vi "Template Test - 24V.vi"(0 "Limits File Path":path, 5 "Results File Path":path, 11 "error in":errorcluster) -> (15 "error out":errorcluster)   [LabVIEW 2024]
doc: "Template test"
uses:
  <vilib>/addons/_JKI Toolkits/State Machine/_JKI_lib_State_Machine.llb/Select State(s)_err__jki_lib_state_machine.vi
  <userlib>/_OpenG.lib/file/file.llb/openg_file.lvlib
  <vilib>/Utility/file.llb/Read Delimited Spreadsheet (string).vi
  <userlib>/_OpenG.lib/file/file.llb/Strip Path Extension - String__ogtk.vi
  <userlib>/_OpenG.lib/appcontrol/appcontrol.llb/openg_application_control.lvlib
  <userlib>/_OpenG.lib/time/time.llb/openg_time.lvlib
  <vilib>/DAQmx/read.llb/DAQmx Read (Digital 1D Bool 1Chan 1Samp).vi
  <vilib>/DAQmx/create/channels.llb/DAQmx Create Channel (DI-Digital Input).vi
  <vilib>/addons/_JKI Toolkits/State Machine/_JKI_lib_State_Machine.llb/Select State(s)_bool__jki_lib_state_machine.vi
  <vilib>/Utility/file.llb/Write Delimited Spreadsheet (string).vi
panel:
  out "Timer Results Data":string[](array[string])
  out "24V Results Data":string[](array[string])
  in  "Exit":bool
  # "LED Test VI"
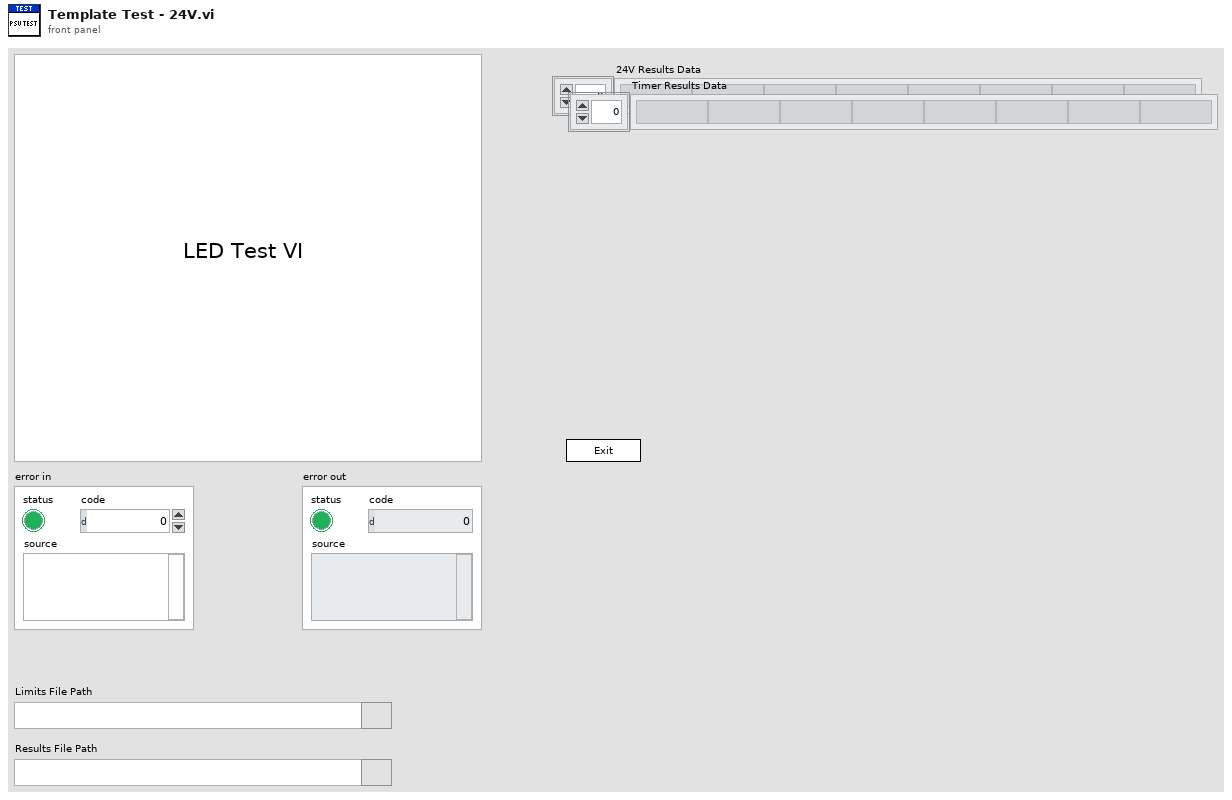
[diagram p1: front panel]
types:
  T1 = enum32{"Invalid", "Standard", "Closed", "Hidden", "Minimized", "Maximized"}
  T2 = enum32{"invalid app kind", "Development System", "Run Time System", "Student Edition", "Embedded LabVIEW", "Evaluation", "Custom"}
  T3 = enum16{"Start Timer", "Get Time", "Pause", "Unpause"}
  T4 = cluster{"Core":cluster{"Current VI Reference":refnum<vi>, "Close Panel on Exit?":bool}, "Limits File Path":path, "Test Limits":string[][], "Results Data Array":string[][], "Results File Path":path, "24V?":bool, "Time Elapsed?":bool, "task out":refnum<k21>}
  T5 = cluster{"Current VI Reference":refnum<vi>, "Close Panel on Exit?":bool}
  T6 = cluster{"[0]":bool, "[1]":bool, "[2]":bool, "[3]":bool, "[4]":bool, "[5]":bool, "[6]":bool, "[7]":bool, "[8]":bool}
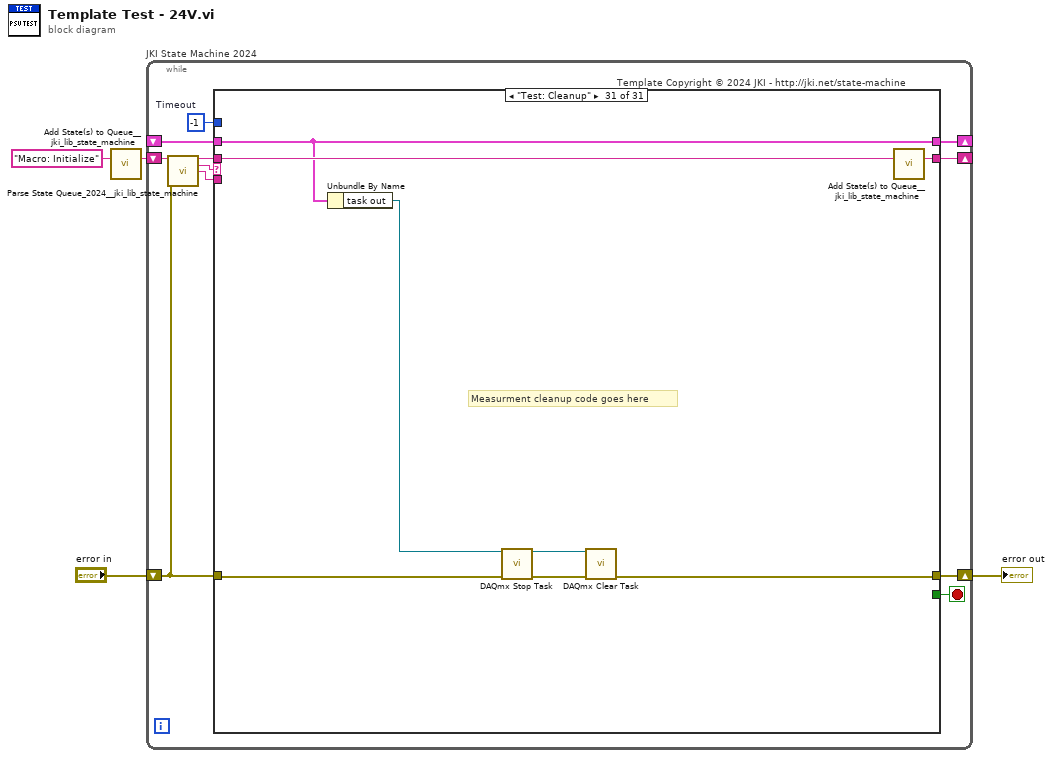
[diagram p0: block diagram]
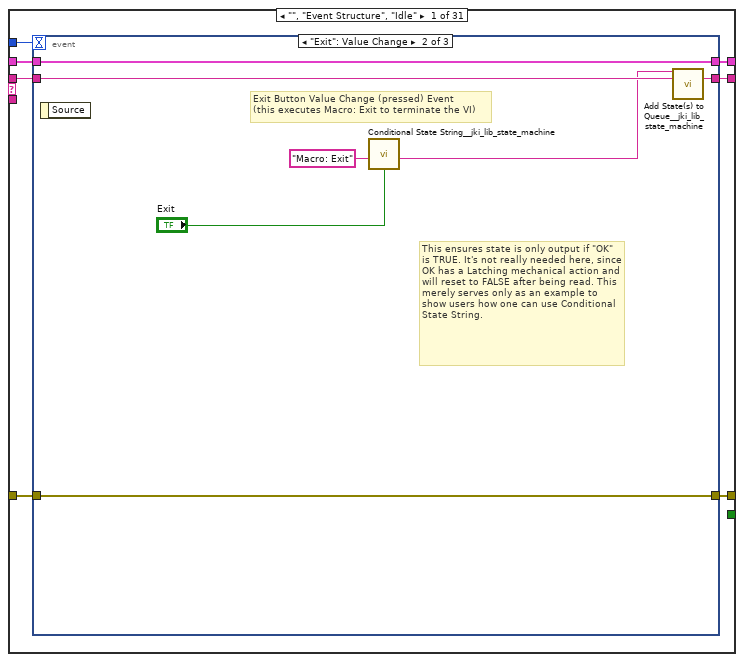
[diagram p2: hidden frame]
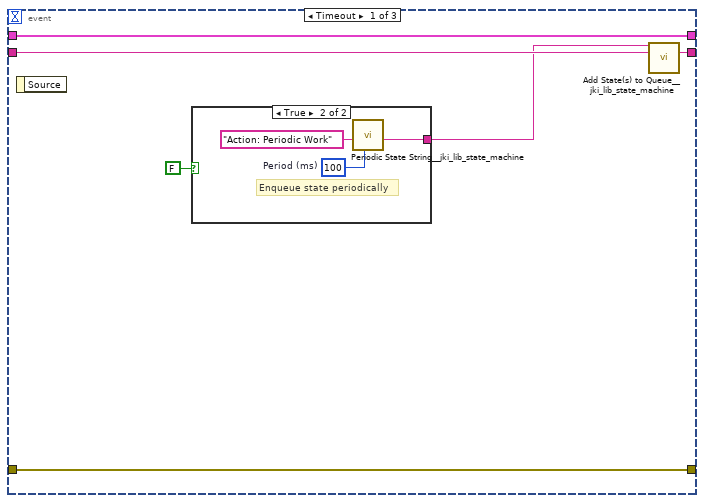
[diagram p3: hidden frame]
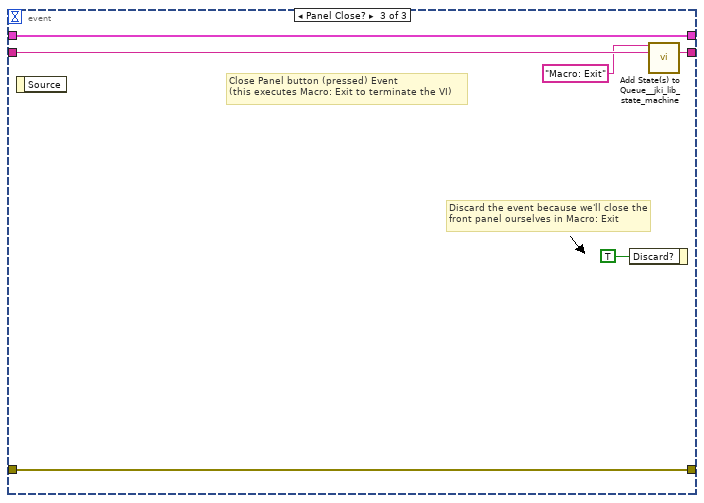
[diagram p5: hidden frame]
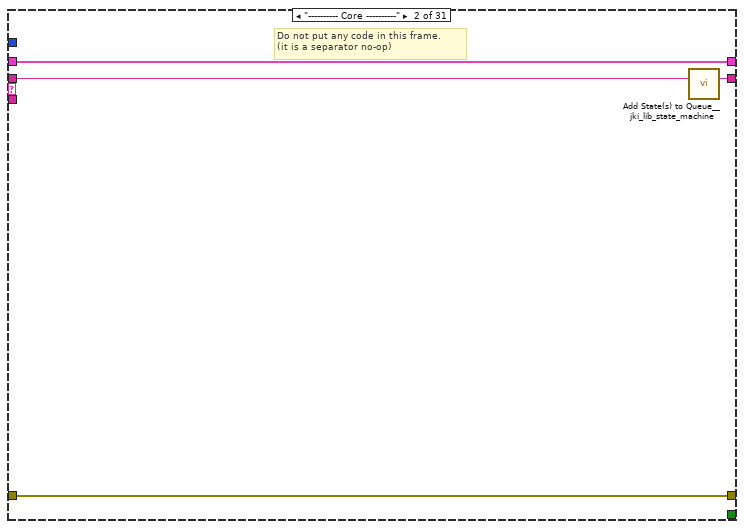
[diagram p6: hidden frame]
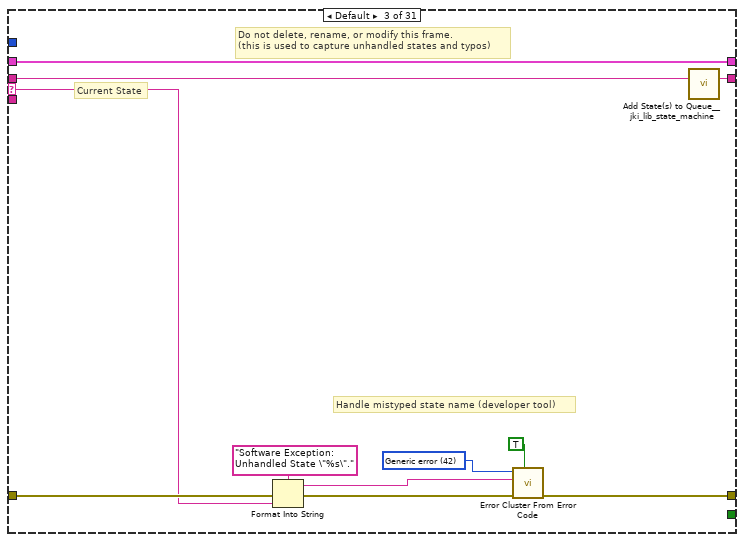
[diagram p7: hidden frame]
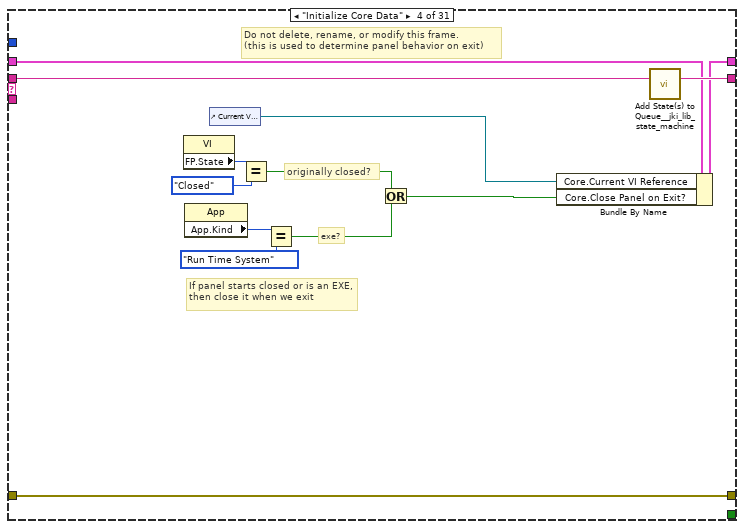
[diagram p8: hidden frame]
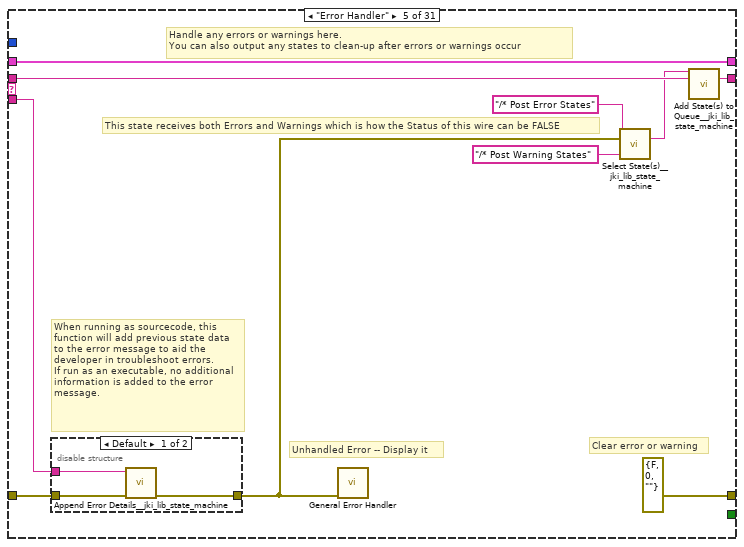
[diagram p9: hidden frame]
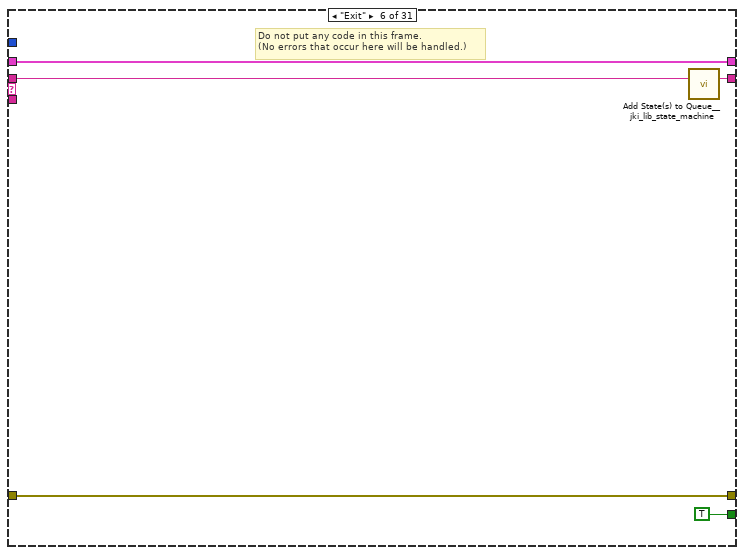
[diagram p11: hidden frame]
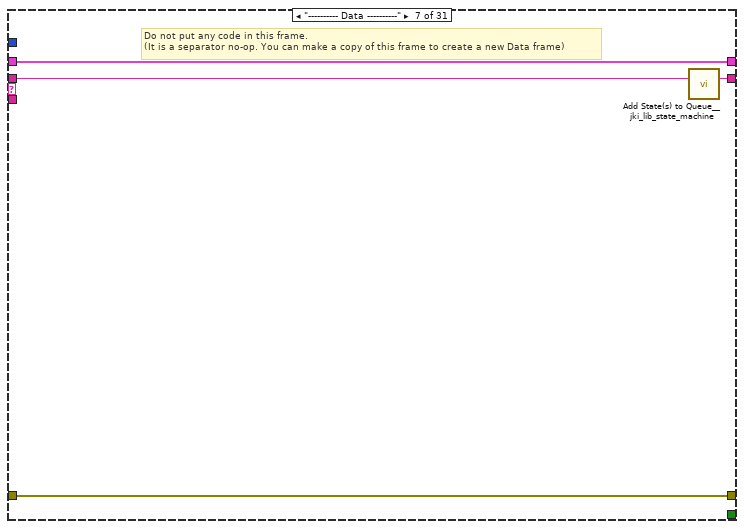
[diagram p12: hidden frame]
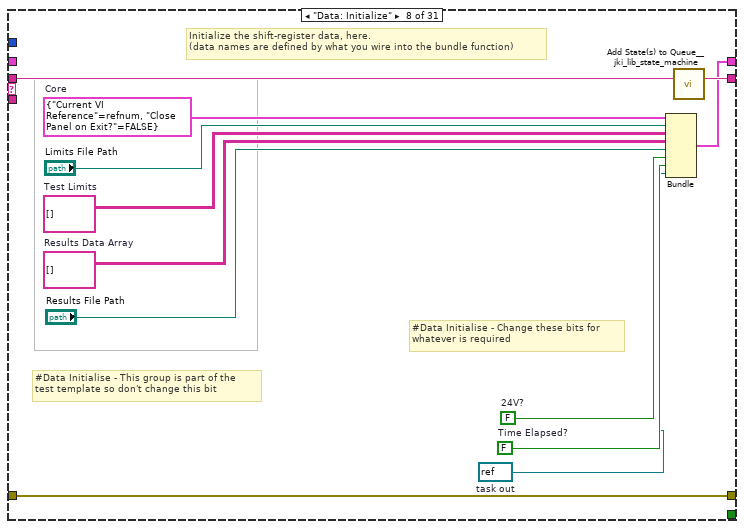
[diagram p13: hidden frame]
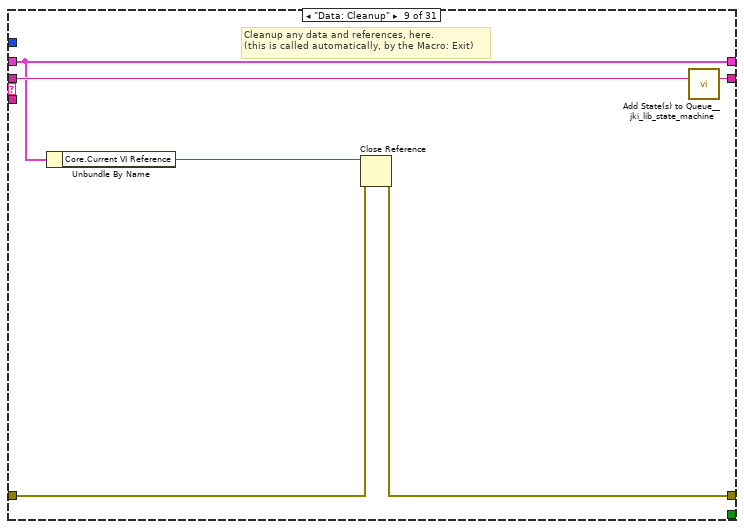
[diagram p14: hidden frame]
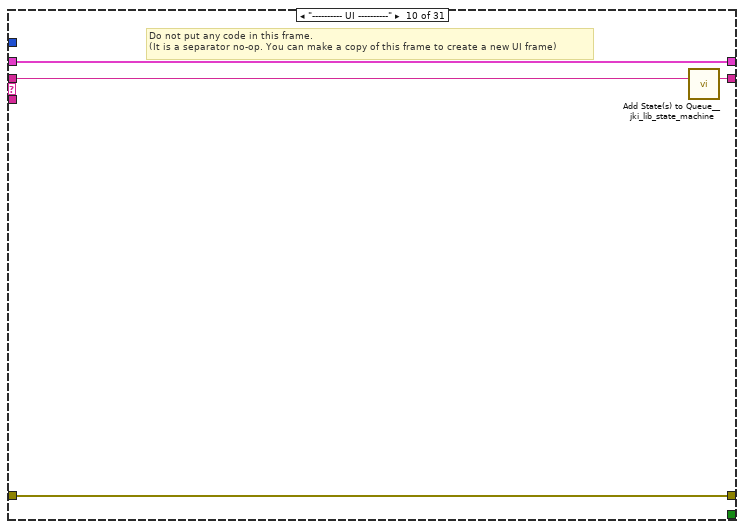
[diagram p15: hidden frame]
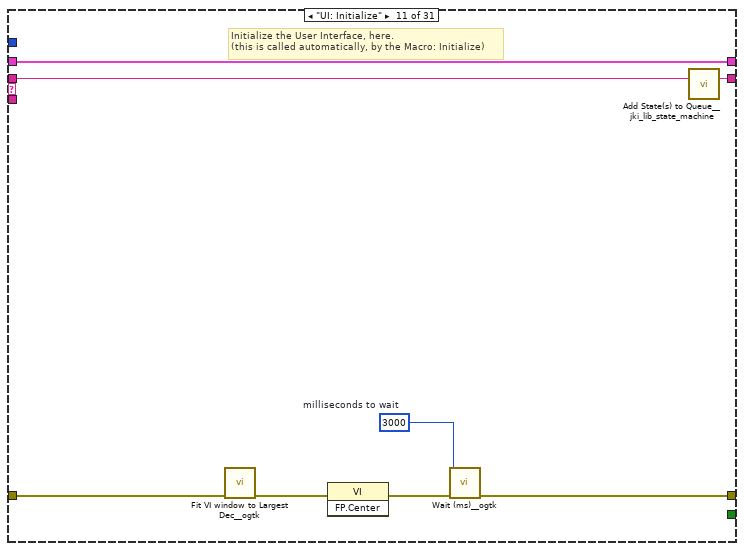
[diagram p16: hidden frame]
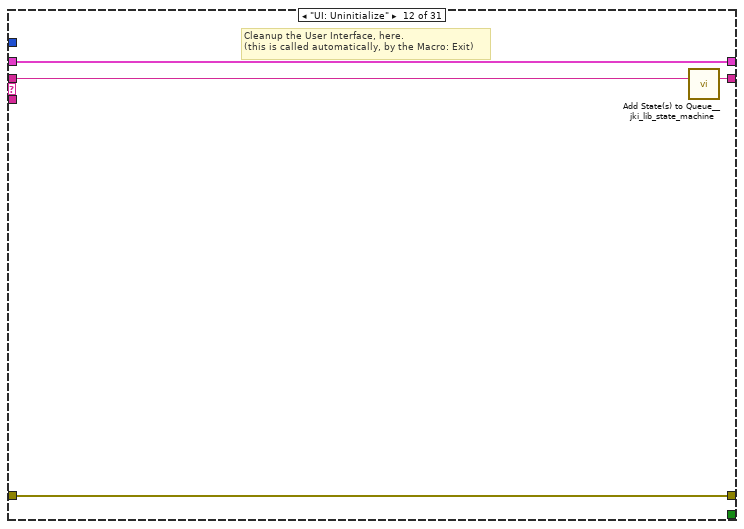
[diagram p17: hidden frame]
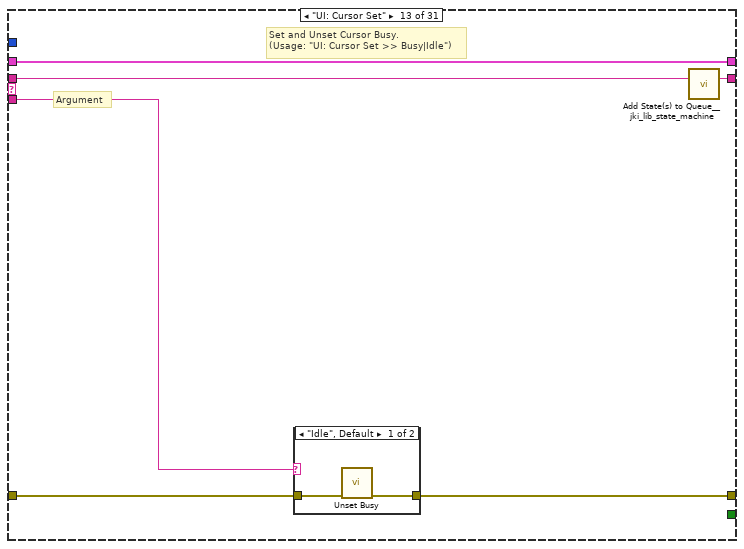
[diagram p18: hidden frame]
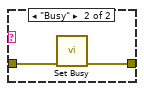
[diagram p19: hidden frame]
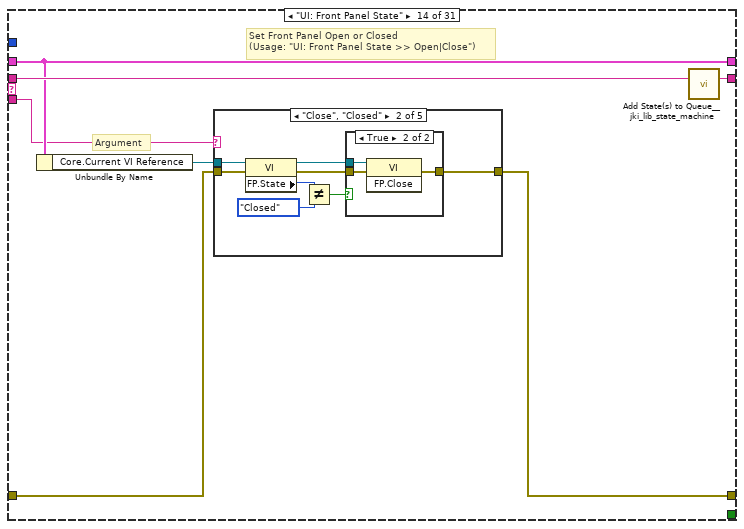
[diagram p20: hidden frame]
diagram:
  n1 = call <vilib>:"Add State(s) to Queue__jki_lib_state_machine.vi"("State(s) in (\"\")"="Macro: Initialize") -> ("States Out"=w4:string)  [unwired: 14 in]
  n2 = while "JKI State Machine 2024" {
    shift-right: [w8] -> _
    shift-left: _ -> [w7]
    shift-right: [w11] -> w1
    shift-left: "error in" -> [w5]
    shift-right: [w10] -> _
    shift-left: w4 -> [w12]
    stop <- w9 stop-if-true
    w6 = -1  # Timeout
    # "Template Copyright © 2024 JKI - http://jki.net/state-machine"
    n3 = call <vilib>:"Parse State Queue_2024__jki_lib_state_machine.vi"("State Queue"=w12, "Error In (no error)"=w5) -> ("Remaining States"=w14:string, "Current State"=w15:string, "Arguments"=w13:string)  [unwired: 11 in]
    n4 = case shown="\"Test: Cleanup\"" w15 {
      selector: w15 -> [_ _ w49 _ _ _ _ _ _ _ _ _ _ _ _ _ _ _ _ _ _ _ _ _ _ _ _ _ _ _ _]
      tunnel: w14 -> [w22 w48 w53 w72 w82 w91 w95 w107 w113 w117 w125 w129 w135 w146 w215 w220 w225 w230 w239 w243 w256 w273 w286 w290 w299 w303 w313 w319 w337 w349 w357]
      tunnel: w13 -> [_ _ _ _ w77 _ _ _ _ _ _ _ w130 w140 _ _ _ _ _ _ _ _ _ _ _ _ _ _ _ _ _]
      tunnel: w7 -> [w20 w45 w51 w65 w79 w89 w92 _ w108 w114 w123 w127 w133 w142 w212 w217 w222 w227 w237 w240 w246 w265 w278 w287 w295 w300 w306 w317 w321 w340 w351]
      tunnel: [w19 w46 w55 w69 errorcluster {"status"=FALSE, "code"=0, "source"=""} ("error out") w88 w93 w104 w109 w115 w121 w126 w131 w143 w213 w218 w223 w228 w234 w241 w252 w270 w283 w288 w297 w301 w307 w314 w326 w345 w353] -> w11
      tunnel: w5 -> [w16 w46 w54 w69 w78 w88 w93 w104 w110 w115 w122 w126 w132 w144 w213 w218 w223 w228 w234 w241 w251 w269 w282 w288 w296 w301 w308 w315 w329 w344 w352]
      tunnel: [w21 w47 w52 w71 w81 w90 w94 w106 w112 w116 w124 w128 w134 w145 w214 w219 w224 w229 w238 w242 w255 w272 w285 w289 w298 w302 w312 w318 w336 w348 w356] -> w10
      tunnel: [_ _ _ _ _ TRUE _ _ _ _ _ _ _ _ _ _ _ _ _ _ _ _ _ _ _ _ _ _ _ _ _] -> w9
      tunnel: [w18 w45 w51 w70 w79 w89 w92 w105 w108 w114 w123 w127 w133 w142 w212 w217 w222 w227 w237 w240 w245 w264 w277 w287 w295 w300 w305 w317 w335 w339 w351] -> w8
      tunnel: w6 -> [w17 _ _ _ _ _ _ _ _ _ _ _ _ _ _ _ _ _ _ _ _ _ _ _ _ _ _ _ _ _ _]
      frame "", "Event Structure", "Idle" {
        n5 = event shown="[1] \"Exit\": Value Change" {
          selector: _ -> [_ _ _]
          dyn-events: _ -> [_ _ _]
          timeout: w17 -> [_ _ _]
          tunnel: w22 -> [w28 w38 w44]
          tunnel: [w27 w37 w43] -> w21
          tunnel: w20 -> [w25 w35 w41]
          tunnel: [w26 w36 w42] -> w19
          tunnel: w16 -> [w26 w36 w42]
          tunnel: [w25 w35 w41] -> w18
          event Timeout {
            n6 = event-data() -> ()  [unwired: 1 in, 1 out]
            n7 = case shown="True" FALSE {
              tunnel: [_ w31] -> w24
              frame False {
              }
              frame True {
                w29 = u32 100  # Period (ms)
                # "Enqueue state periodically"
                n8 = call <vilib>:"Periodic State String__jki_lib_state_machine.vi"("Period (ms)"=w29, "State"="Action: Periodic Work") -> ("State Out"=w31:string)  [unwired: 9 in]
              }
            }
            n9 = call <vilib>:"Add State(s) to Queue__jki_lib_state_machine.vi"("State(s) in Front (\"\")"=w24, "State(s) in (\"\")"=w28) -> ("States Out"=w27:string)  [unwired: 13 in]
          }
          event "Exit": Value Change {
            # "This ensures state is only output if \"OK\" is TRUE. It's not really needed here, since OK has a Latching mechanical action and will reset to FALSE after being read. This merely serves only as an example to show users how one can use Conditional State String."
            # "Exit Button Value Change (pressed) Event\n(this executes Macro: Exit to terminate the VI)"
            n10 = event-data() -> ()  [unwired: 1 in, 1 out]
            n11 = call <vilib>:"Conditional State String__jki_lib_state_machine.vi"("Do State(s)?"="Exit", "State"="Macro: Exit") -> ("State Out"=w32:string)  [unwired: 7 in]
            n12 = call <vilib>:"Add State(s) to Queue__jki_lib_state_machine.vi"("State(s) in Front (\"\")"=w32, "State(s) in (\"\")"=w38) -> ("States Out"=w37:string)  [unwired: 13 in]
          }
          event Panel Close? {
            # "Discard the event because we'll close the front panel ourselves in Macro: Exit"
            # "Close Panel button (pressed) Event\n(this executes Macro: Exit to terminate the VI)"
            n13 = event-data() -> ()  [unwired: 1 in, 1 out]
            n14 = event-data("Discard?"=TRUE) -> ()  [unwired: 1 in, 1 out]
            n15 = call <vilib>:"Add State(s) to Queue__jki_lib_state_machine.vi"("State(s) in Front (\"\")"="Macro: Exit", "State(s) in (\"\")"=w44) -> ("States Out"=w43:string)  [unwired: 13 in]
          }
        }
      }
      frame "---------- Core ----------" {
        # "Do not put any code in this frame.\n(it is a separator no-op)"
        n16 = call <vilib>:"Add State(s) to Queue__jki_lib_state_machine.vi"("State(s) in (\"\")"=w48) -> ("States Out"=w47:string)  [unwired: 14 in]
      }
      frame Default {
        w58 = 42 items=["No error", "Argument error", "Memory is full", "Out of zone", "End of file", "File already open", "Generic file I/O error", "File not found", "File permission error", "Disk is full", "Duplicate path", "Too many files open", "System feature not enabled", "Resource file not found", "Cannot add resource", "Resource not found", "Image not found", "Image memory error", "Pen does not exist", "Config type invalid", "Config token not found", "Config parse error", "Config memory error", "Bad external code format", "Bad external code offset", "External code not present", "Null window", "Destroy window error", "Null menu", "Print aborted", "Bad print record", "Print driver error", "Windows error during printing", "Memory error during printing", "Print dialog error", "Generic print error", "Invalid device refnum", "Device not found", "Device parameter error", "Device unit error", "Cannot open device", "Device call aborted", "Generic error", "Cancelled by user", "Object ID too low", "Object ID too high", "Object not in heap", "Unknown heap", "Unknown object (invalid DefProc)", "Unknown object (DefProc not in table)", "Message out of range", "Invalid (null) method", "Unknown message", "Manager call not supported", "Bad address", "Network operation in progress", "Network operation timed out", "Connection is busy", "Network attribute not supported", "Network error", "Address in use", "System out of memory", "Connection aborted", "Connection refused", "Not connected", "Already connected", "Connection closed", "Initialization error (interapplication manager)", "Bad occurrence", "Wait on unbound occurrence handler", "Occurrence queue overflow", "Datalog type conflict", "Unused", "Unrecognized type (interapplication manager)", "Memory corrupt", "Failed to make temporary DLL", "Old CIN version", "Drag socket not found", "Failed to load drop-object", "Failed to register OLE object", "Failed to release OLE object", "Format specifier type mismatch", "Unknown format specifier", "Too few format specifiers", "Too many format specifiers", "Scan failed", "Newer CIN version", "Error converting to variant", "Runtime menu error", "Password tampered", "Variant attribute not found", "Incompatible variant data type", "Event data is not available", "Event Store is not present", "Occurrence is not found", "Event Queue is not created", "Event info is not available", "Refnum passed is NULL", "Error retrieving Class GUID", "Error retrieving CoClass GUID", "Error retrieving TypeLib GUID.", "Bad built application magic bytes.", "Specific driver is different from the specific driver associated with the Logical Name.", "There is no session opened to the class driver.", "Max Error", "MAX - Error with config objects", "MAX - Error loading configuration", "MAX - Group not supported"]
        # "Current State"
        # "Do not delete, rename, or modify this frame.\n(this is used to capture unhandled states and typos)"
        # "Handle mistyped state name (developer tool)"
        n17 = Format Into String(format string="Software Exception: Unhandled State \"%s\"." ("message"), error in=w54, w49) -> (resulting string=w57:string, error out=w56:errorcluster)  [unwired: 1 in]
        n18 = call <vilib>:"Error Cluster From Error Code.vi"("show call chain? (False)"=TRUE, "error in (no error)"=w56, "error message (\"\")"=w57, "error code (0)"=w58) -> ("error out"=w55:errorcluster)  [unwired: 5 in]
        n19 = call <vilib>:"Add State(s) to Queue__jki_lib_state_machine.vi"("State(s) in (\"\")"=w53) -> ("States Out"=w52:string)  [unwired: 14 in]
      }
      frame "Initialize Core Data" {
        # "Do not delete, rename, or modify this frame.\n(this is used to determine panel behavior on exit)"
        # "originally closed?"
        # "exe?"
        # "If panel starts closed or is an EXE, then close it when we exit"
        n20 = property class="VI"() -> ("FP.State"=w62:T1)  [unwired: 2 in, 2 out]
        n21 = property class="App"() -> ("App.Kind"=w68:T2)  [unwired: 2 in, 2 out]
        n22 = control-ref of="Current VI Reference"() -> (w63:refnum<vi>)
        n23 = Equal?(x=w62, y=T1."Closed" ("Front Panel Window:State")) -> (x = y?=w60:bool)
        n24 = Equal?(x=w68, y=T2."Run Time System" ("Application:Kind")) -> (x = y?=w66:bool)
        n25 = Or(x=w60, y=w66) -> (x .or. y?=w64:bool)
        n26 = Bundle By Name(cluster=w65, "Core.Current VI Reference"=w63, "Core.Close Panel on Exit?"=w64) -> (w70:T4)
        n27 = call <vilib>:"Add State(s) to Queue__jki_lib_state_machine.vi"("State(s) in (\"\")"=w72) -> ("States Out"=w71:string)  [unwired: 14 in]
      }
      frame "Error Handler" {
        # "When running as sourcecode, this function will add previous state data to the error message to aid the developer in troubleshoot errors.\nIf run as an executable, no additional information is added to the error message."
        # "This state receives both Errors and Warnings which is how the Status of this wire can be FALSE"
        # "Unhandled Error -- Display it"
        # "Handle any errors or warnings here.\nYou can also output any states to clean-up after errors or warnings occur"
        # "Clear error or warning"
        n28 = disable-structure shown="Default" {
          disable-tunnel: w78 -> [w85 w86]
          disable-tunnel: w77 -> [w84 _]
          disable-tunnel: [w83 w86] -> w76
          frame condition #0 (active) {
            n29 = call <vilib>:"Append Error Details__jki_lib_state_machine.vi"("error in (no error)"=w85, "Previous State and Argument(s)"=w84) -> ("error out"=w83:errorcluster)  [unwired: 9 in]
          }
          frame condition #1 {
          }
        }
        n30 = call <vilib>:"General Error Handler.vi"("error in (no error)"=w76) -> ()  [unwired: 10 in, 5 out]
        n31 = call-poly <vilib>:"Select State(s)__jki_lib_state_machine.vi"("State(s) if True (\"\")"="/* Post Error States", "Select"=w76, "State(s) if False (\"\")"="/* Post Warning States") -> ("States Out"=w74:string)  [unwired: 12 in]
        n32 = call <vilib>:"Add State(s) to Queue__jki_lib_state_machine.vi"("State(s) in Front (\"\")"=w74, "State(s) in (\"\")"=w82) -> ("States Out"=w81:string)  [unwired: 13 in]
      }
      frame "Exit" {
        # "Do not put any code in this frame.\n(No errors that occur here will be handled.)"
        n33 = call <vilib>:"Add State(s) to Queue__jki_lib_state_machine.vi"("State(s) in (\"\")"=w91) -> ("States Out"=w90:string)  [unwired: 14 in]
      }
      frame "---------- Data ----------" {
        # "Do not put any code in this frame.\n(It is a separator no-op. You can make a copy of this frame to create a new Data frame)"
        n34 = call <vilib>:"Add State(s) to Queue__jki_lib_state_machine.vi"("State(s) in (\"\")"=w95) -> ("States Out"=w94:string)  [unwired: 14 in]
      }
      frame "Data: Initialize" {
        w96 = refnum<k21> refnum  # task out
        w97 = FALSE  # Time Elapsed?
        w98 = FALSE  # 24V?
        w100 = string[][] []  # Results Data Array
        w101 = string[][] []  # Test Limits
        w103 = T5 {"Current VI Reference"=refnum, "Close Panel on Exit?"=FALSE}  # Core
        # "#Data Initialise - Change these bits for\nwhatever is required"
        # "#Data Initialise - This group is part of the\ntest template so don't change this bit"
        # "Initialize the shift-register data, here.\n(data names are defined by what you wire into the bundle function)"
        n35 = Bundle("Core"=w103, "Limits File Path"="Limits File Path", "Test Limits"=w101, "Results Data Array"=w100, "Results File Path"="Results File Path", "24V?"=w98, "Time Elapsed?"=w97, "task out"=w96) -> (w105:T4)  [unwired: 1 in]
        n36 = call <vilib>:"Add State(s) to Queue__jki_lib_state_machine.vi"("State(s) in (\"\")"=w107) -> ("States Out"=w106:string)  [unwired: 14 in]
      }
      frame "Data: Cleanup" {
        # "Cleanup any data and references, here.\n(this is called automatically, by the Macro: Exit)"
        n37 = Unbundle By Name(w108) -> ("Core.Current VI Reference"=w111:refnum<vi>)
        n38 = Close Reference(reference=w111, error in (no error)=w110) -> (error out=w109:errorcluster)
        n39 = call <vilib>:"Add State(s) to Queue__jki_lib_state_machine.vi"("State(s) in (\"\")"=w113) -> ("States Out"=w112:string)  [unwired: 14 in]
      }
      frame "---------- UI ----------" {
        # "Do not put any code in this frame.\n(It is a separator no-op. You can make a copy of this frame to create a new UI frame)"
        n40 = call <vilib>:"Add State(s) to Queue__jki_lib_state_machine.vi"("State(s) in (\"\")"=w117) -> ("States Out"=w116:string)  [unwired: 14 in]
      }
      frame "UI: Initialize" {
        w120 = u32 3000  # milliseconds to wait
        # "Initialize the User Interface, here.\n(this is called automatically, by the Macro: Initialize)"
        n41 = call <userlib>:"Fit VI window to Largest Dec__ogtk.vi"("error in (no error)"=w122) -> ("error out"=w118:errorcluster)  [unwired: 5 in, 1 out]
        n42 = invoke class="VI" method="FP.Center"(error in=w118) -> (error out=w119:errorcluster)  [unwired: 2 in, 2 out]
        n43 = call <userlib>:"Wait (ms)__ogtk.vi"("error in (no error)"=w119, "milliseconds to wait"=w120) -> ("error out"=w121:errorcluster)  [unwired: 8 in, 1 out]
        n44 = call <vilib>:"Add State(s) to Queue__jki_lib_state_machine.vi"("State(s) in (\"\")"=w125) -> ("States Out"=w124:string)  [unwired: 14 in]
      }
      frame "UI: Uninitialize" {
        # "Cleanup the User Interface, here.\n(this is called automatically, by the Macro: Exit)"
        n45 = call <vilib>:"Add State(s) to Queue__jki_lib_state_machine.vi"("State(s) in (\"\")"=w129) -> ("States Out"=w128:string)  [unwired: 14 in]
      }
      frame "UI: Cursor Set" {
        # "Argument"
        # "Set and Unset Cursor Busy.\n(Usage: \"UI: Cursor Set >> Busy|Idle\")"
        n46 = case shown="\"Idle\", Default" w130 {
          tunnel: w132 -> [w137 w139]
          tunnel: [w136 w138] -> w131
          frame "Idle", Default {
            n47 = call <vilib>:"Unset Busy.vi"("error in (no error)"=w137) -> ("error out"=w136:errorcluster)  [unwired: 10 in]
          }
          frame "Busy" {
            n48 = call <vilib>:"Set Busy.vi"("error in (no error)"=w139) -> ("error out"=w138:errorcluster)  [unwired: 9 in, 1 out]
          }
        }
        n49 = call <vilib>:"Add State(s) to Queue__jki_lib_state_machine.vi"("State(s) in (\"\")"=w135) -> ("States Out"=w134:string)  [unwired: 14 in]
      }
      frame "UI: Front Panel State" {
        # "Argument"
        # "Set Front Panel Open or Closed\n(Usage: \"UI: Front Panel State >> Open|Close\")"
        n50 = Unbundle By Name(w142) -> ("Core.Current VI Reference"=w141:refnum<vi>)
        n51 = case shown="\"Close\", \"Closed\"" w140 {
          tunnel: w144 -> [w152 w167 w178 w191 w204]
          tunnel: [w154 w168 w180 w193 w206] -> w143
          tunnel: w141 -> [w153 w165 w179 w192 w205]
          frame "Open", "Standard", Default {
            w147 = T1."Standard" ("State")
            n52 = property class="VI"(reference=w153, error in=w152) -> (reference out=w150:refnum<vi>, error out=w151:errorcluster, "FP.State"=w149:T1)
            n53 = Not Equal?(x=w149, y=w147) -> (x != y?=w148:bool)
            n54 = case shown="True" w148 {
              tunnel: [w158 w160] -> w154
              tunnel: w151 -> [w157 w160]
              tunnel: w150 -> [w156 _]
              tunnel: w147 -> [w155 _]
              frame True {
                n55 = invoke class="VI" method="FP.Open"(reference=w156, error in=w157, "Activate"=TRUE, "State"=w155) -> (error out=w158:errorcluster)  [unwired: 1 in, 4 out]
              }
              frame False {
              }
            }
          }
          frame "Close", "Closed" {
            n56 = property class="VI"(reference=w165, error in=w167) -> (reference out=w164:refnum<vi>, error out=w166:errorcluster, "FP.State"=w162:T1)
            n57 = Not Equal?(x=w162, y=T1."Closed" ("Front Panel Window:State")) -> (x != y?=w161:bool)
            n58 = case shown="True" w161 {
              tunnel: [w169 w172] -> w168
              tunnel: w166 -> [w169 w171]
              tunnel: w164 -> [_ w170]
              frame False {
              }
              frame True {
                n59 = invoke class="VI" method="FP.Close"(reference=w170, error in=w171) -> (error out=w172:errorcluster)  [unwired: 1 in, 2 out]
              }
            }
          }
          frame "Hidden", "Hide" {
            w173 = T1."Hidden" ("State")
            n60 = property class="VI"(reference=w179, error in=w178) -> (reference out=w176:refnum<vi>, error out=w177:errorcluster, "FP.State"=w175:T1)
            n61 = Not Equal?(x=w175, y=w173) -> (x != y?=w174:bool)
            n62 = case shown="True" w174 {
              tunnel: [w184 w185] -> w180
              tunnel: w177 -> [w183 w185]
              tunnel: w176 -> [w182 _]
              tunnel: w173 -> [w181 _]
              frame True {
                n63 = invoke class="VI" method="FP.Open"(reference=w182, error in=w183, "State"=w181) -> (error out=w184:errorcluster)  [unwired: 2 in, 4 out]
              }
              frame False {
              }
            }
          }
          frame "Minimize", "Minimized" {
            w186 = T1."Minimized" ("State")
            n64 = property class="VI"(reference=w192, error in=w191) -> (reference out=w189:refnum<vi>, error out=w190:errorcluster, "FP.State"=w188:T1)
            n65 = Not Equal?(x=w188, y=w186) -> (x != y?=w187:bool)
            n66 = case shown="True" w187 {
              tunnel: [w197 w198] -> w193
              tunnel: w190 -> [w196 w198]
              tunnel: w189 -> [w195 _]
              tunnel: w186 -> [w194 _]
              frame True {
                n67 = invoke class="VI" method="FP.Open"(reference=w195, error in=w196, "State"=w194) -> (error out=w197:errorcluster)  [unwired: 2 in, 4 out]
              }
              frame False {
              }
            }
          }
          frame "Maximize", "Maximized" {
            w199 = T1."Maximized" ("State")
            n68 = property class="VI"(reference=w205, error in=w204) -> (reference out=w202:refnum<vi>, error out=w203:errorcluster, "FP.State"=w201:T1)
            n69 = Not Equal?(x=w201, y=w199) -> (x != y?=w200:bool)
            n70 = case shown="True" w200 {
              tunnel: [w210 w211] -> w206
              tunnel: w203 -> [w209 w211]
              tunnel: w202 -> [w208 _]
              tunnel: w199 -> [w207 _]
              frame True {
                n71 = invoke class="VI" method="FP.Open"(reference=w208, error in=w209, "State"=w207) -> (error out=w210:errorcluster)  [unwired: 2 in, 4 out]
              }
              frame False {
              }
            }
          }
        }
        n72 = call <vilib>:"Add State(s) to Queue__jki_lib_state_machine.vi"("State(s) in (\"\")"=w146) -> ("States Out"=w145:string)  [unwired: 14 in]
      }
      frame "---------- Macro ----------" {
        # "Do not put any code in this frame.\n(It is a separator no-op. You can make a copy of this frame to create a new Macro frame)"
        n73 = call <vilib>:"Add State(s) to Queue__jki_lib_state_machine.vi"("State(s) in (\"\")"=w215) -> ("States Out"=w214:string)  [unwired: 14 in]
      }
      frame "Macro: Initialize" {
        # "Initialization Macro\n(This is called once, when the VI starts)"
        n74 = call <vilib>:"Add State(s) to Queue__jki_lib_state_machine.vi"("State(s) in Front (\"\")"="Data: Initialize\nInitialize Core Data\nUI: Initialize\nUI: Front Panel State >> Open\nMacro: Test", "State(s) in (\"\")"=w220) -> ("States Out"=w219:string)  [unwired: 13 in]
      }
      frame "Macro: Test" {
        # "#Test Macro - Add the sequence \nfor measurments and limits testing here"
        n75 = call <vilib>:"Add State(s) to Queue__jki_lib_state_machine.vi"("State(s) in Front (\"\")"="Test: Initialise\nTest: Start Timer\nTest: Measurment", "State(s) in (\"\")"=w225) -> ("States Out"=w224:string)  [unwired: 13 in]
      }
      frame "Macro: Limits" {
        # "#Test Macro - Add the sequence \nfor measurments and limits testing here"
        n76 = call <vilib>:"Add State(s) to Queue__jki_lib_state_machine.vi"("State(s) in Front (\"\")"="Limits Test: Read Limits File\nLimits Test: 24V Test\nLimits Test: Timer Elapsed\nMacro: Exit", "State(s) in (\"\")"=w230) -> ("States Out"=w229:string)  [unwired: 13 in]
      }
      frame "Macro: Exit" {
        # "Exit Macro\n(This is called once, when the VI exits)"
        n77 = Unbundle By Name(w237) -> ("Core.Close Panel on Exit?"=w232:bool)
        n78 = call <vilib>:"Conditional State String__jki_lib_state_machine.vi"("Do State(s)?"=w232, "State"="UI: Front Panel State >> Close") -> ("State Out"=w231:string)  [unwired: 7 in]
        n79 = call <vilib>:"Add State(s) to Queue__jki_lib_state_machine.vi"("State(s) in (\"\")"=w231, "State(s) at Back (\"\")"="Test: Cleanup\nUI: Uninitialize\nData: Cleanup\nExit") -> ("States Out"=w235:string)  [unwired: 13 in]
        n80 = call <vilib>:"Add State(s) to Queue__jki_lib_state_machine.vi"("State(s) in Front (\"\")"=w235, "State(s) in (\"\")"=w239) -> ("States Out"=w238:string)  [unwired: 13 in]
      }
      frame "---------- Limits Test ----------" {
        # "Template Separator\n(You can make a copy of, or modify, this frame)"
        n81 = call <vilib>:"Add State(s) to Queue__jki_lib_state_machine.vi"("State(s) in (\"\")"=w243) -> ("States Out"=w242:string)  [unwired: 14 in]
      }
      frame "Limits Test: Read Limits File" {
        w249 = ","  # delimiter (\t)
        n82 = Unbundle By Name(w246) -> ("Limits File Path"=w250:path)
        n83 = Current VI's Path "Test Case Path"() -> (path=w254:path)
        n84 = call-poly <vilib>:"Read Delimited Spreadsheet.vi"("file path (dialog if empty)"=w250, "error in (no error)"=w251, "delimiter (\\t)"=w249) -> ("all rows"=w247:string[][], "error out"=w252:errorcluster)  [unwired: 7 in, 4 out]
        n85 = Strip Path(path=w254) -> (name=w253:string)  [unwired: 1 out]
        n86 = call-poly <userlib>:"Strip Path Extension__ogtk.vi"("path"=w253) -> ("root"=w248:string)  [unwired: 1 out]
        n87 = for {
          tunnel: w248 -> [w260]
          tunnel: w247 -> [w258] mode=indexing
          tunnel: [w258] -> w244 mode=indexing if=w257
          n88 = Index Array(array=w258) -> (element=w259:string)  [unwired: 1 in]
          n89 = Equal?(x=w260, y=w259) -> (x = y?=w257:bool)
        }
        n90 = Bundle By Name(cluster=w246, "Test Limits"=w244) -> (w245:T4)
        n91 = call <vilib>:"Add State(s) to Queue__jki_lib_state_machine.vi"("State(s) in (\"\")"=w256) -> ("States Out"=w255:string)  [unwired: 14 in]
      }
      frame "Limits Test: 24V Test" {
        w266 = "24V Test"  # Sub Test Name
        # "#Limits Testing - Add the sub test name for\ntest included in limits file"
        n92 = Unbundle By Name(w265) -> ("Results Data Array"=w263:string[][])
        n93 = Unbundle By Name(w265) -> ("Test Limits"=w267:string[][], "24V?"=w271:bool)
        n94 = To Variant(anything=w271) -> (Variant=w268:variant)
        n95 = call "Process Results.vi"("error in (no error)"=w269, "Measurment"=w268, "Test Limits"=w267, "Sub Test Name"=w266) -> ("error out"=w270:errorcluster, "Results Data"=w262:string[])  [unwired: 6 in]
        "24V Results Data" <- w262
        n96 = Build Array (concatenate)(w263, w262) -> (w261:string[][])
        n97 = Bundle By Name(cluster=w265, "Results Data Array"=w261) -> (w264:T4)
        n98 = call <vilib>:"Add State(s) to Queue__jki_lib_state_machine.vi"("State(s) in (\"\")"=w273) -> ("States Out"=w272:string)  [unwired: 14 in]
      }
      frame "Limits Test: Timer Elapsed" {
        w279 = "TimerTest"  # Sub Test Name
        # "#Limits Testing - Add the sub test name for\ntest included in limits file"
        n99 = Unbundle By Name(w278) -> ("Test Limits"=w280:string[][], "Time Elapsed?"=w284:bool)
        n100 = Unbundle By Name(w278) -> ("Results Data Array"=w276:string[][])
        n101 = To Variant(anything=w284) -> (Variant=w281:variant)
        n102 = call "Process Results.vi"("error in (no error)"=w282, "Measurment"=w281, "Test Limits"=w280, "Sub Test Name"=w279) -> ("error out"=w283:errorcluster, "Results Data"=w275:string[])  [unwired: 6 in]
        "Timer Results Data" <- w275
        n103 = Build Array (concatenate)(w276, w275) -> (w274:string[][])
        n104 = Bundle By Name(cluster=w278, "Results Data Array"=w274) -> (w277:T4)
        n105 = call <vilib>:"Add State(s) to Queue__jki_lib_state_machine.vi"("State(s) in (\"\")"=w286) -> ("States Out"=w285:string)  [unwired: 14 in]
      }
      frame "---------- Results Data ----------" {
        # "Template Separator\n(You can make a copy of, or modify, this frame)"
        n106 = call <vilib>:"Add State(s) to Queue__jki_lib_state_machine.vi"("State(s) in (\"\")"=w290) -> ("States Out"=w289:string)  [unwired: 14 in]
      }
      frame "Results Data: Write Results Data" {
        w291 = ","  # delimiter (\t)
        w292 = TRUE  # append to file? (new file:F)
        n107 = Unbundle By Name(w295) -> ("Results File Path"=w294:path, "Results Data Array"=w293:string[][])
        n108 = call-poly <vilib>:"Write Delimited Spreadsheet.vi"("file path (dialog if empty)"=w294, "2D data"=w293, "append to file? (new file:F)"=w292, "error in (no error)"=w296, "delimiter (\\t)"=w291) -> ("error out"=w297:errorcluster)  [unwired: 9 in, 1 out]
        n109 = call <vilib>:"Add State(s) to Queue__jki_lib_state_machine.vi"("State(s) in (\"\")"=w299) -> ("States Out"=w298:string)  [unwired: 14 in]
      }
      frame "---------- Test ----------" {
        # "Template Separator\n(You can make a copy of, or modify, this frame)"
        n110 = call <vilib>:"Add State(s) to Queue__jki_lib_state_machine.vi"("State(s) in (\"\")"=w303) -> ("States Out"=w302:string)  [unwired: 14 in]
      }
      frame "Test: Initialise" {
        # "Measurement initialisation code goes here"
        n111 = call-poly <vilib>:"DAQmx Create Virtual Channel.vi"("lines"=tag "6525/port1", "error in"=w308) -> ("task out"=w311:refnum<k21>, "error out"=w310:errorcluster)  [unwired: 12 in]
        n112 = call <vilib>:"DAQmx Start Task.vi"("task/channels in"=w311, "error in"=w310) -> ("task out"=w304:refnum<k21>, "error out"=w307:errorcluster)  [unwired: 12 in]
        n113 = Bundle By Name(cluster=w306, "task out"=w304) -> (w305:T4)
        n114 = call <vilib>:"Add State(s) to Queue__jki_lib_state_machine.vi"("State(s) in (\"\")"=w313) -> ("States Out"=w312:string)  [unwired: 14 in]
      }
      frame "Test: Start Timer" {
        # "Template Separator\n(You can make a copy of, or modify, this frame)"
        n115 = call "Timer.vi"("error in (no error)"=w315, "Enum"=T3."Start Timer") -> ("error out"=w314:errorcluster)  [unwired: 6 in, 3 out]
        n116 = call <vilib>:"Add State(s) to Queue__jki_lib_state_machine.vi"("State(s) in (\"\")"=w319) -> ("States Out"=w318:string)  [unwired: 14 in]
      }
      frame "Test: Measurment" {
        # "Measurment Code here"
        n117 = Unbundle By Name(w321) -> ("task out"=w320:refnum<k21>)
        n118 = call-poly <vilib>:"DAQmx Read.vi"("task/channels in"=w320, "error in"=w329) -> ("data"=w328:bool[], "error out"=w326:errorcluster)  [unwired: 11 in, 1 out]
        n119 = Equal?(x=bool[] [TRUE, TRUE, TRUE], y=w328) -> (x = y?=w334:bool[])
        n120 = Array To Cluster(array=w334) -> (cluster=w333:T6)
        n121 = Unbundle(w333) -> ("[0]"=w332:bool, "[1]"=w331:bool, "[2]"=w330:bool)  [unwired: 6 out]
        n122 = Compound Arithmetic op=AND(w332, w331, w330) -> (w325:bool)
        n123 = Bundle By Name(cluster=w321, "24V?"=w325) -> (w335:T4)
        n124 = call-poly <vilib>:"Select State(s)__jki_lib_state_machine.vi"("State(s) if True (\"\")"="Macro: Limits" ("State(s) if True (\"\")"), "Select"=w325, "State(s) if False (\"\")"="Test: Elapsed Timer" ("State(s) if False (\"\")")) -> ("States Out"=w322:string)  [unwired: 12 in]
        n125 = call <vilib>:"Add State(s) to Queue__jki_lib_state_machine.vi"("State(s) in Front (\"\")"=w322, "State(s) in (\"\")"=w337) -> ("States Out"=w336:string)  [unwired: 13 in]
      }
      frame "Test: Elapsed Timer" {
        # "Template Separator\n(You can make a copy of, or modify, this frame)"
        n126 = call "Timer.vi"("error in (no error)"=w344, "Target Time"=3.0, "Enum"=T3."Get Time") -> ("error out"=w345:errorcluster, "Time Elapsed?"=w338:bool)  [unwired: 5 in, 2 out]
        n127 = Bundle By Name(cluster=w340, "Time Elapsed?"=w338) -> (w339:T4)
        n128 = call-poly <vilib>:"Select State(s)__jki_lib_state_machine.vi"("State(s) if True (\"\")"="Limits Test: 24V Test" ("State(s) if True (\"\")"), "Select"=w338, "State(s) if False (\"\")"="Test: Measurment" ("State(s) if False (\"\")")) -> ("States Out"=w341:string)  [unwired: 12 in]
        n129 = call <vilib>:"Add State(s) to Queue__jki_lib_state_machine.vi"("State(s) in Front (\"\")"=w341, "State(s) in (\"\")"=w349) -> ("States Out"=w348:string)  [unwired: 13 in]
      }
      frame "Test: Cleanup" {
        # "Measurment cleanup code goes here"
        n130 = Unbundle By Name(w351) -> ("task out"=w350:refnum<k21>)
        n131 = call <vilib>:"DAQmx Stop Task.vi"("task/channels in"=w350, "error in"=w352) -> ("task out"=w354:refnum<k21>, "error out"=w355:errorcluster)  [unwired: 12 in]
        n132 = call <vilib>:"DAQmx Clear Task.vi"("task in"=w354, "error in"=w355) -> ("error out"=w353:errorcluster)  [unwired: 13 in]
        n133 = call <vilib>:"Add State(s) to Queue__jki_lib_state_machine.vi"("State(s) in (\"\")"=w357) -> ("States Out"=w356:string)  [unwired: 14 in]
      }
    }
  }
  "error out" <- w1
